vi "SRX_Config Set Slot CL Values.vi"(6 "Send Cmd Timout(ms)":u32, 7 "SlotIdx":i32, 8 "Error":errorcluster, 9 "CL":T1 {"Gains"."F" format="%#.8f"; "Gains"."D" format="%#.8f"; "Gains"."I" format="%#.8f"; "Gains"."P" format="%#.8f"}, 11 "PhoenixMotorControlDevRef":T3) -> (0 "Error Out":errorcluster, 1 "CL Out":T1 {"Gains"."F" format="%#.8f"; "Gains"."D" format="%#.8f"; "Gains"."I" format="%#.8f"; "Gains"."P" format="%#.8f"}, 3 "PhoenixMotorControlDevRef Out":T3)   [LabVIEW 2023]
uses:
  Shared Code/TypeDefs/Cluster_SRX SLOT PID Config.ctl
  Shared Code/TypeDefs/Cluster_PID Gains.ctl
  <vilib>/Rock Robotics/WPI/MotorControl/WPI_MotorControlDeviceRef.ctl
  <vilib>/Rock Robotics/WPI/MotorControl/WPI_MotorControlType.ctl
  <vilib>/Rock Robotics/SystemInterfaces/DIO/FPGA_DIOPWMChannel.ctl
  <vilib>/Rock Robotics/WPI/PWM/WPI_PWMDeadband.ctl
  <vilib>/Rock Robotics/SystemInterfaces/DIO/FPGA_DIOChannel.ctl
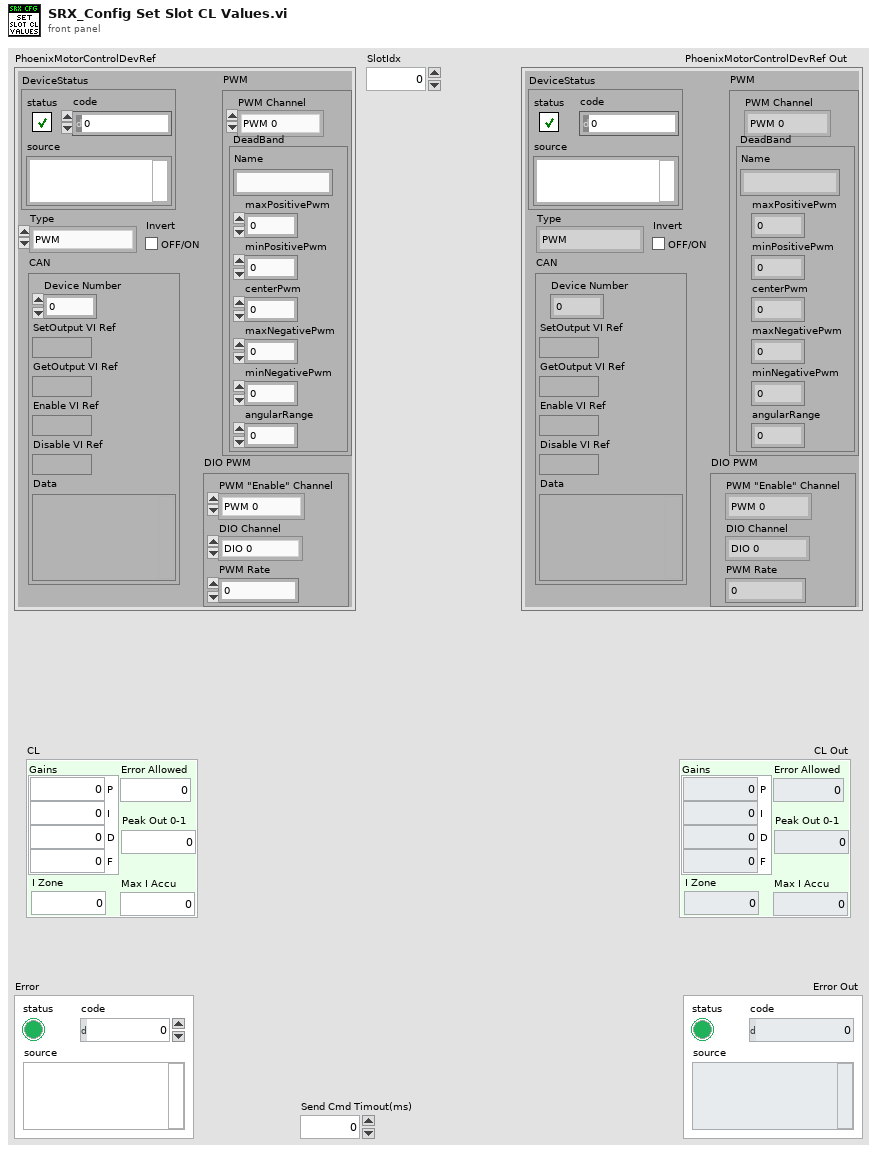
[diagram p1: front panel]
types:
  T1 = typedef "Cluster_SRX SLOT PID Config.ctl" = cluster{"Gains":T2, "Error Allowed":dbl, "I Zone":dbl, "Peak Out 0-1":dbl, "Max I Accu":dbl}
  T2 = typedef "Cluster_PID Gains.ctl" = cluster{"P":dbl, "I":dbl, "D":dbl, "F":dbl}
  T3 = typedef "WPI_MotorControlDeviceRef.ctl" = cluster{"DeviceStatus":errorcluster, "Type":T4, "PWM":cluster{"PWM Channel":T5, "DeadBand":T6}, "CAN":cluster{"Device Number":u8, "SetOutput VI Ref":variant, "GetOutput VI Ref":variant, "Enable VI Ref":variant, "Disable VI Ref":variant, "Data":variant}, "Invert":bool, "DIO PWM":cluster{"PWM \"Enable\" Channel":T5, "DIOChannel":T7, "PWM Rate":dbl}}
  T4 = typedef "WPI_MotorControlType.ctl" = enum16{"PWM", "CAN", "DIO PWM"}
  T5 = typedef "FPGA_DIOPWMChannel.ctl" = enum8{"PWM 0", "PWM 1", "PWM 2", "PWM 3", "PWM 4", "PWM 5", "PWM 6", "PWM 7", "PWM 8", "PWM 9", "PWM MXP 0", "PWM MXP 1", "PWM MXP 2", "PWM MXP 3", "PWM MXP 4", "PWM MXP 5", "PWM MXP 6", "PWM MXP 7", "PWM MXP 8", "PWM MXP 9", "Invalid"}
  T6 = typedef "WPI_PWMDeadband.ctl" = cluster{"Name":string, "maxPositivePwm":i32, "minPositivePwm":i32, "centerPwm":i32, "maxNegativePwm":i32, "minNegativePwm":i32, "angularRange":u16}
  T7 = typedef "FPGA_DIOChannel.ctl" = enum8{"DIO 0", "DIO 1", "DIO 2", "DIO 3", "DIO 4", "DIO 5", "DIO 6", "DIO 7", "DIO 8", "DIO 9", "DIO MXP 0", "DIO MXP 1", "DIO MXP 2", "DIO MXP 3", "DIO MXP 4", "DIO MXP 5", "DIO MXP 6", "DIO MXP 7", "DIO MXP 8", "DIO MXP 9", "DIO MXP 10", "DIO MXP 11", "DIO MXP 12", "DIO MXP 13", "DIO MXP 14", "DIO MXP 15", "SPI Port CS1", "SPI Port CS2", "SPI Port CS3", "SPI Port MISO", "SPI Port MOSI", "Invalid"}
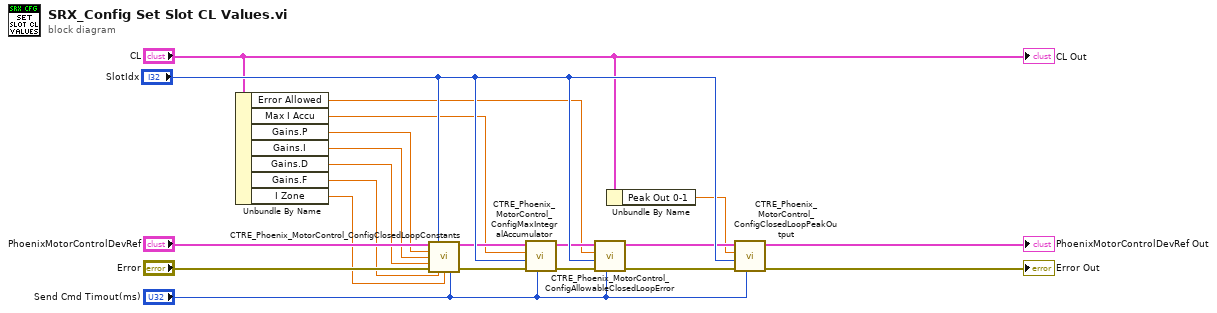
[diagram p0: block diagram]
diagram:
  n1 = Unbundle By Name("CL") -> ("Error Allowed"=w7:dbl, "Max I Accu"=w6:dbl, "Gains.P"=w12:dbl, "Gains.I"=w11:dbl, "Gains.D"=w10:dbl, "Gains.F"=w9:dbl, "I Zone"=w8:dbl)
  n2 = call <vilib>:"CTRE_Phoenix_MotorControl_ConfigClosedLoopConstants.vi"("PhoenixMotorControlDevRef"="PhoenixMotorControlDevRef", "slotIdx"="SlotIdx", "P"=w12, "I"=w11, "D"=w10, "error in (no error)"="Error", "F"=w9, "I Zone"=w8, "timeoutMs"="Send Cmd Timout(ms)") -> ("PhoenixMotorControlDevRef"=w13:T3, "error out"=w15:errorcluster)  [unwired: 5 in]
  n3 = call <vilib>:"CTRE_Phoenix_MotorControl_ConfigMaxIntegralAccumulator.vi"("timeoutMs"="Send Cmd Timout(ms)", "error in (no error)"=w15, "slotIdx"="SlotIdx", "Maximum Integral Accumulator Value"=w6, "PhoenixMotorControlDevRef"=w13) -> ("error out"=w16:errorcluster, "PhoenixMotorControlDevRef"=w14:T3)  [unwired: 5 in]
  n4 = call <vilib>:"CTRE_Phoenix_MotorControl_ConfigAllowableClosedLoopError.vi"("timeoutMs"="Send Cmd Timout(ms)", "error in (no error)"=w16, "slotIdx"="SlotIdx", "allowableClosedLoopError"=w7, "PhoenixMotorControlDevRef"=w14) -> ("error out"=w4:errorcluster, "PhoenixMotorControlDevRef"=w5:T3)  [unwired: 5 in]
  n5 = Unbundle By Name("CL") -> ("Peak Out 0-1"=w3:dbl)
  n6 = call <vilib>:"CTRE_Phoenix_MotorControl_ConfigClosedLoopPeakOutput.vi"("timoutMs"="Send Cmd Timout(ms)", "error in (no error)"=w4, "slotIdx"="SlotIdx", "peakOutput"=w3, "PhoenixMotorControlDevRef"=w5) -> ("error out"=→"Error Out":errorcluster, "PhoenixMotorControlDevRef"=→"PhoenixMotorControlDevRef Out":T3)  [unwired: 5 in]
  "CL Out" <- "CL"
